vi "Solution Write Low Level.vi"(8 "error in (no error)":errorcluster, 9 "Author ID":i32, 10 "Layer Information Cluster":T1 {"Deposition Method" items=["Front Electrode", "Electron Transport Layer", "Active Layer", "Hole Transport Layer", "Back Electrode", "Custom Layer"]; "Layer Type" items=["Front Electrode", "Electron Transport Layer", "Active Layer", "Hole Transport Layer", "Back Electrode", "Custom Layer"]}, 11 "Database Connection In":T2) -> (0 "error out":errorcluster, 3 "Database Connection Out":T2)   [LabVIEW 2020]
uses:
  <vilib>/addons/database/Connection.llb/Conn ObjectReference.ctl
  Data Clusters/Layer Information Cluster.ctl
  <vilib>/addons/database/NI_Database_API.lvlib
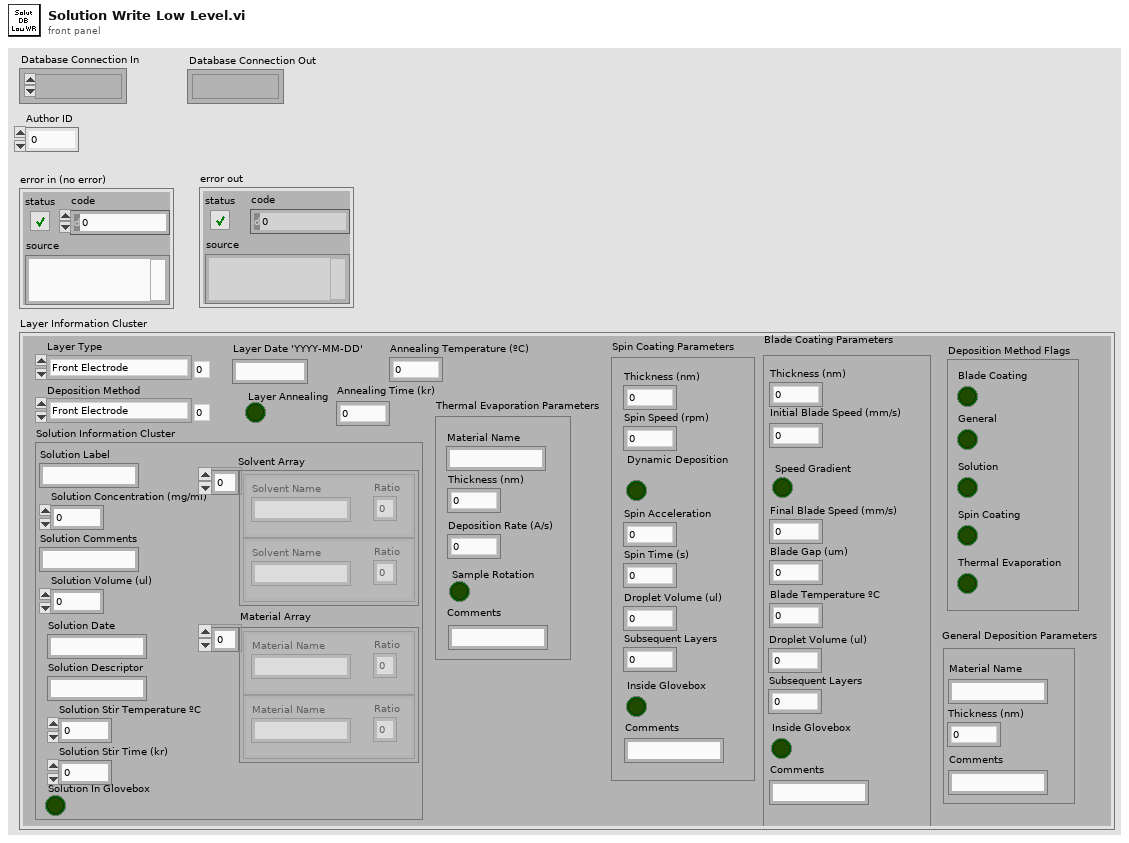
[diagram p1: front panel]
types:
  T1 = typedef "Layer Information Cluster.ctl" = cluster{"Solution Information Cluster":cluster{"Solution Label":string, "Solution Concentration (mg/ml)":dbl, "Solution Comments ":string, "Solution Volume (ul) ":dbl, "Solution Date ":string, "Solution Descriptor ":string, "Solution Stir Temperature ºC ":dbl, "Solution Stir Time (kr) ":dbl, "Solution In Glovebox":bool, "Solvent Array":cluster{"Solvent Name":string, "Ratio":dbl}[], "Material Array":cluster{"Material Name":string, "Ratio":dbl}[]}, "Layer Type":u16, "Deposition Method":u16, "Layer Annealing":bool, "General Deposition Parameters":cluster{"Thickness (nm)":dbl, "Comments":string, "Material Name":string}, "Blade Coating Parameters":cluster{"Thickness (nm)":dbl, "Initial Blade Speed (mm/s)":dbl, "Speed Gradient":bool, "Final Blade Speed (mm/s)":dbl, "Blade Gap (um)":dbl, "Droplet Volume (ul)":dbl, "Subsequent Layers":dbl, "Inside Glovebox":bool, "Comments":string, "Blade Temperature ºC":dbl}, "Spin Coating Parameters":cluster{"Thickness (nm)":dbl, "Spin Speed (rpm)":dbl, "Dynamic Deposition":bool, "Spin Acceleration":dbl, "Spin Time (s)":dbl, "Droplet Volume (ul)":dbl, "Subsequent Layers":dbl, "Inside Glovebox":bool, "Comments":string}, "Thermal Evaporation Parameters":cluster{"Deposition Rate (A/s)":dbl, "Thickness (nm)":dbl, "Comments":string, "Material Name":string, "Sample Rotation":bool}, "Layer Date 'YYYY-MM-DD'":string, "Annealing Time (kr)":dbl, "Annealing Temperature (ºC)":dbl, "Deposition Method Flags":cluster{"Blade Coating":bool, "General ":bool, "Solution":bool, "Spin Coating":bool, "Thermal Evaporation":bool}}
  T2 = typedef "NI_Database_API.lvlib/Conn ObjectReference.ctl" = refnum<k1>
  T3 = cluster{"Solution Label":string, "Solution Concentration (mg/ml)":dbl, "Solution Volume (ul) ":dbl, "Solution Stir Temperature ºC ":dbl, "Solution Stir Time (kr) ":dbl, "Solution Date ":string, "Solution In Glovebox":bool, "Solution Comments ":string, "Solution Descriptor ":string, "Author ID":i32}
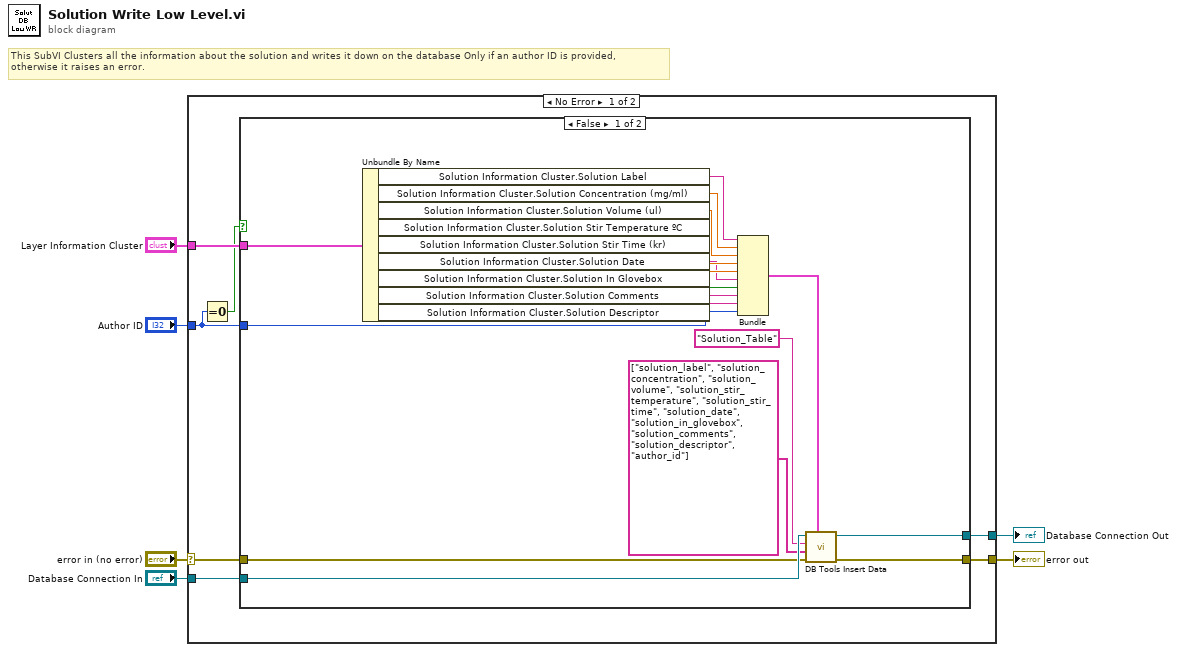
[diagram p0: block diagram]
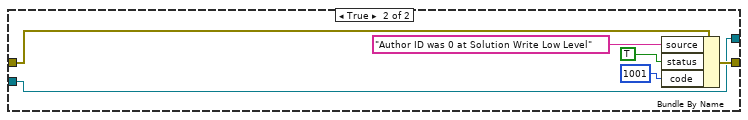
[diagram p2: hidden frame]
diagram:
  # "This SubVI Clusters all the information about the solution and writes it down on the database Only if an author ID is provided,\notherwise it raises an error."
  n1 = case shown="No Error" "error in (no error)" {
    selector: "error in (no error)" -> [w10 w38]
    tunnel: [w13 w38] -> w6
    tunnel: [w12 w39] -> w5
    tunnel: "Database Connection In" -> [w11 w39]
    tunnel: "Layer Information Cluster" -> [w9 _]
    tunnel: "Author ID" -> [w8 _]
    frame No Error {
      n2 = Equal To 0?(x=w8) -> (x = 0?=w7:bool)
      n3 = case shown="False" w7 {
        tunnel: [w31 w34] -> w13
        tunnel: [w30 w33] -> w12
        tunnel: w11 -> [w29 w33]
        tunnel: w10 -> [w28 w32]
        tunnel: w9 -> [w26 _]
        tunnel: w8 -> [w17 _]
        frame False {
          n4 = Unbundle By Name(w26) -> ("Solution Information Cluster.Solution Label"=w23:string, "Solution Information Cluster.Solution Concentration (mg/ml)"=w22:dbl, "Solution Information Cluster.Solution Volume (ul)"=w21:dbl, "Solution Information Cluster.Solution Stir Temperature ºC"=w20:dbl, "Solution Information Cluster.Solution Stir Time (kr)"=w19:dbl, "Solution Information Cluster.Solution Date"=w14:string, "Solution Information Cluster.Solution In Glovebox"=w18:bool, "Solution Information Cluster.Solution Comments"=w25:string, "Solution Information Cluster.Solution Descriptor"=w24:string)
          n5 = Bundle("Solution Label"=w23, "Solution Concentration (mg/ml)"=w22, "Solution Volume (ul)"=w21, "Solution Stir Temperature ºC"=w20, "Solution Stir Time (kr)"=w19, "Solution Date"=w14, "Solution In Glovebox"=w18, "Solution Comments"=w25, "Solution Descriptor"=w24, "Author ID"=w17) -> (w16:T3)  [unwired: 1 in]
          n6 = call <vilib>:"DB Tools Insert Data.vi"("data"=w16, "error in (no error)"=w28, "columns"=string[] ["solution_label", "solution_concentration", "solution_volume", "solution_stir_temperature", "solution_stir_time", "solution_date", "solution_in_glovebox", "solution_comments", "solution_descriptor", "author_id"], "table"="Solution_Table", "connection reference"=w29) -> ("error out"=w31:errorcluster, "connection reference out"=w30:T2)  [unwired: 5 in]
        }
        frame True {
          n7 = Bundle By Name(cluster=w32, "source"="Author ID was 0 at Solution Write Low Level", "status"=TRUE, "code"=1001) -> (w34:errorcluster)
        }
      }
    }
    frame Error {
    }
  }
  "error out" <- w6
  "Database Connection Out" <- w5
